vi "GregorianCal_MonthLengths.vi"(10 "Year (0: this year)":i32) -> (2 "Month Lengths":i32[](array[numeric]))   [LabVIEW 2018]
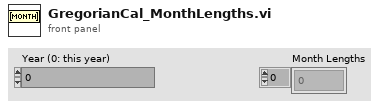
[diagram p1: front panel]
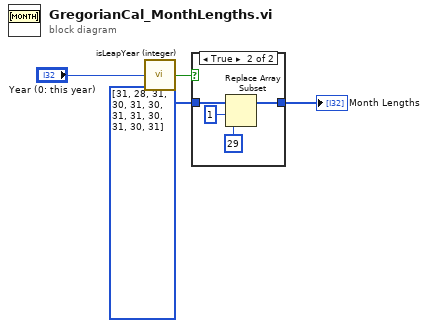
[diagram p0: block diagram]
diagram:
  n1 = call "isLeapYear (integer).vi"("Year (0: this year)"="Year (0: this year)") -> ("is Leap Year?"=w2:bool)  [unwired: 8 in]
  n2 = case shown="True" w2 {
    tunnel: i32[] [31, 28, 31, 30, 31, 30, 31, 31, 30, 31, 30, 31] -> [w5 w9]
    tunnel: [w5 w6] -> w3
    frame False {
    }
    frame True {
      n3 = Replace Array Subset(array=w9, new element=29 ("value"), index=1) -> (w6:i32[])
    }
  }
  "Month Lengths" <- w3
